vi "EdgeDetector.vi"(1 "DetectorType":T1, 2 "Input":bool) -> (0 "Edge":bool)   [LabVIEW 2017, in "ArgosLib.lvlib"]
uses:
  ArgosLib.lvlib
  TypeDefs/EdgeDetector_Type.ctl
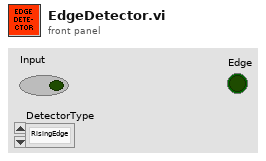
[diagram p1: front panel]
types:
  T1 = typedef "ArgosLib.lvlib/EdgeDetector_Type.ctl" = enum16{"RisingEdge", "FallingEdge", "Both"}
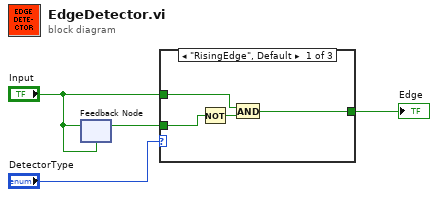
[diagram p0: block diagram]
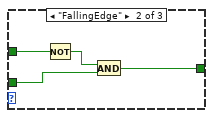
[diagram p2: hidden frame]
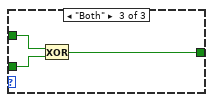
[diagram p3: hidden frame]
diagram:
  n1 = feedback-in #1("Input") -> ()
  n2 = feedback #1("Input") -> (w2:bool)
  n3 = case shown="\"RisingEdge\", Default" "DetectorType" {
    tunnel: "Input" -> [w8 w11 w15]
    tunnel: w2 -> [w6 w10 w14]
    tunnel: [w5 w9 w13] -> w1
    frame "RisingEdge", Default {
      n4 = Not(x=w6) -> (.not. x?=w7:bool)
      n5 = And(x=w8, y=w7) -> (x .and. y?=w5:bool)
    }
    frame "FallingEdge" {
      n6 = Not(x=w11) -> (.not. x?=w12:bool)
      n7 = And(x=w12, y=w10) -> (x .and. y?=w9:bool)
    }
    frame "Both" {
      n8 = Exclusive Or(1:w14, 2:w15) -> (0:w13:bool)
    }
  }
  "Edge" <- w1
